vi "Update frame period global.vi"(8 "error in (no error)":errorcluster) -> (0 "error out":errorcluster)   [LabVIEW 2017]
uses:
  Globals/gl_Time series viewer globals.vi
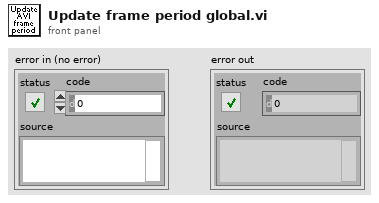
[diagram p1: front panel]
types:
  T1 = typedef "AVI playback header info cluster.ctl" = cluster{"Frame Size":u32, "AOD fill time (us)":dbl, "Dwell time (us)":dbl, "Frame period (ms)":dbl, "Number of Miniscans":u16, "Number of Pixels in Miniscan":u16}
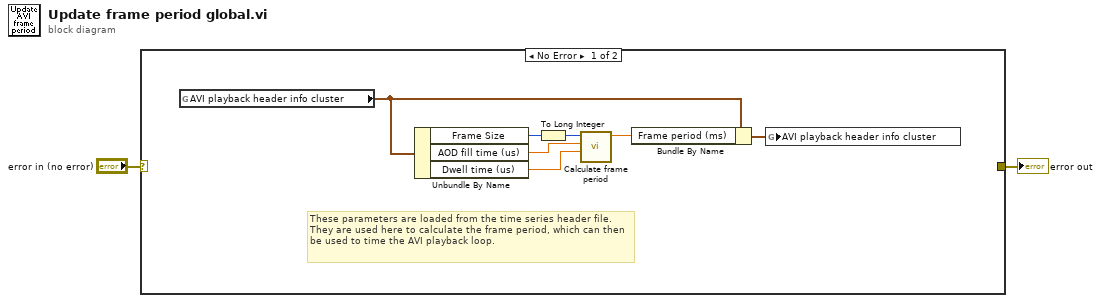
[diagram p0: block diagram]
diagram:
  n1 = case shown="No Error" "error in (no error)" {
    selector: "error in (no error)" -> [_ w10]
    tunnel: [_ w10] -> w1
    frame No Error {
      # "These parameters are loaded from the time series header file.\nThey are used here to calculate the frame period, which can then be used to time the AVI playback loop."
      n2 = global read "gl_Time series viewer globals.vi" "AVI playback header info cluster"() -> (w7:T1)
      n3 = Unbundle By Name(w7) -> ("Frame Size"=w6:u32, "AOD fill time (us)"=w4:dbl, "Dwell time (us)"=w5:dbl)
      n4 = To Long Integer(number=w6) -> (32bit integer=w3:i32)
      n5 = call "Calculate frame period.vi"("Dwell time (us)"=w5, "AOD fill time (us)"=w4, "Frame size (pixels in single dimension)"=w3) -> ("Frame period (ms)"=w8:dbl)  [unwired: 8 in]
      n6 = Bundle By Name(cluster=w7, "Frame period (ms)"=w8) -> (w9:T1)
      n7 = global write "gl_Time series viewer globals.vi" "AVI playback header info cluster"(w9) -> ()
    }
    frame Error {
    }
  }
  "error out" <- w1
